vi "FPGACANTest.vi"   [LabVIEW 2018]
uses:
  <vilib>/FPGAPlugInAG/cRIO-9063/niLvFpga_Open_cRIO-9063.vi
  <vilib>/rvi/interface/common/dynamic/niFpgaDynamicAddResources.vi
  <vilib>/FPGAPlugInAG/Dynamic/niLvFpga_Run_Dynamic.vi
  <vilib>/FPGAPlugInAG/Dynamic/niLvFpga_Abort_Dynamic.vi
  <vilib>/FPGAPlugInAG/Dynamic/niLvFpga_Close_Dynamic.vi
  <vilib>/rvi/interface/nirviOpenFPGA/nirviOpenFPGA.xnode
  FPGA Bitfiles/2019HyperXiteCom_FPGATarget_Fail-SafeControl_eg2p2q-h5Jg.lvbitx
  <vilib>/rvi/interface/nirviMethod/nirviMethod.xnode
  <vilib>/rvi/interface/nirviCloseFPGA/nirviCloseFPGA.xnode
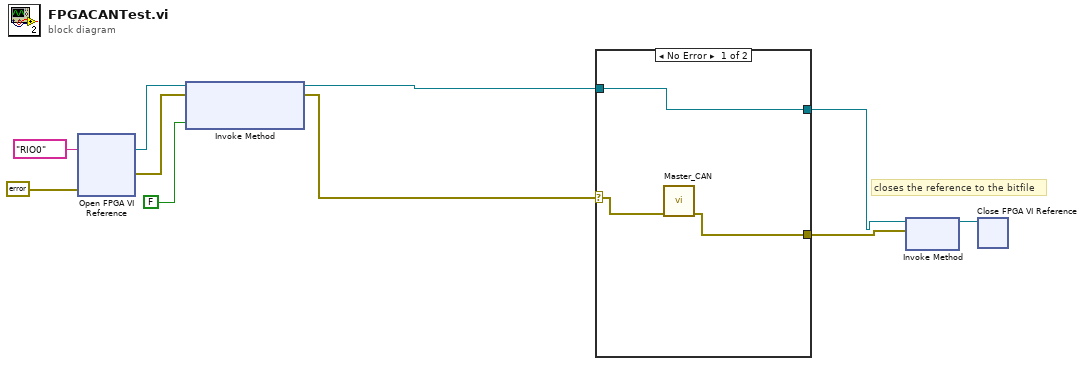
[diagram p0: block diagram]
diagram:
  # "closes the reference to the bitfile"
  n1 = xnode "Open FPGA VI Reference"("error in"=errorcluster {"status"=FALSE, "code"=0, "source"=""}, "resource name"=tag "RIO0") -> ("FPGA VI Reference Out"=w7:refnum<k20>, "error out"=w9:errorcluster)
  n2 = xnode "Invoke Method"("FPGA VI Reference In"=w7, "error in"=w9, "Wait Until Done (F)"=FALSE) -> ("FPGA VI Reference Out"=w2:refnum<k20>, "error out"=w4:errorcluster)
  n3 = case shown="No Error" w4 {
    selector: w4 -> [w12 w14]
    tunnel: [w13 w15] -> w3
    tunnel: w2 -> [w13 w15]
    tunnel: [w11 w14] -> w1
    frame No Error {
      n4 = call "Master_CAN.vi"("error in"=w12) -> ("error out"=w11:errorcluster)  [unwired: 10 in]
    }
    frame Error {
    }
  }
  n5 = xnode "Invoke Method"("FPGA VI Reference In"=w3, "error in"=w1) -> ("FPGA VI Reference Out"=w5:refnum<k20>)  [unwired: 1 out]
  n6 = xnode "Close FPGA VI Reference"("FPGA VI Reference In"=w5) -> ()  [unwired: 1 in, 1 out]
